vi "MIU_Control_v1.3.vi"() -> ()   [LabVIEW 2010]
uses:
  <vilib>/Utility/error.llb/DialogType.ctl
  <vilib>/Instr/_visa.llb/VISA Configure Serial Port (Instr).vi
  <vilib>/Analysis/NI_AALPro.lvlib
panel:
  in  "Tab Control":T1(tab)=enum."Concentrations"
  in  "Serial Read Port":refnum<visa-resource-name>="COM5"
  in  "data bits":u16=8 min=5 max=8 step=1
  in  "parity":u16(ring) items=["None", "Odd", "Even", "Mark", "Space"]
  in  "stop bits":u16(ring)=10 items=["1.0"=10, "1.5"=15, "2.0"=20]
  in  "flow control":u16(ring) items=["None"=0, "XON/XOFF"=1, "RTS/CTS"=2, "DTR/DSR"=4]
  in  "delay before read (ms)":u32=500
  in  "byte count":u32=500
  out "Incoming Serial String":string="    02/28/13 05:18:49.492,    3.20644e-01,    0.00000e+00,    3.33105e-01,    0.00000e+00,    5.19723e+02,    0.00000e+00,    3.20811e-01,    0.00000e+00,    3.33278e-01,    0.00000e+00,    8.02680e+01,    0.00000e+00,    3.33389e+01,    0.00000e+00,    2.71783e+01,    0.00000e+00,    3.55973e-01,    0.00000e+00,    6.31022e-01,    0.00000e+00,    1.95007e+00,    0.00000e+00,              3\n"
  out "Time":string="05:18:49.492"
  out "Date":string="02/28/13"
  out "return count":u32=394
  in  "Instrument baud rate (9600)":u32=9600
  in  "Control Port":refnum<visa-resource-name>="COM4"
  in  "Control baud rate":u32=9600
  out "N2O is FLAT":bool
  out "Rolling CO Slope Fit":cluster{i32[], "Best Linear Fit":dbl[]}[](graph)=[{[0, 1, 2, 3, 4, 5, 6, 7, 8, 9, 10, 11, 12, 13, 14, 15, 16, 17, 18, 19], "Best Linear Fit"=[0.320611, 0.320505, 0.320476, 0.3208, 0.320926, 0.320701, 0.320587, 0.320889, 0.320914, 0.320439, 0.3209, 0.320794, 0.320847, 0.320592, 0.320735, 0.32085, 0.320821, 0.320729, 0.320589, 0.320309]}, {[0, 1, 2, 3, 4, 5, 6, 7, 8, 9, 10, 11, 12, 13, 14, 15, 16, 17, 18, 19], "Best Linear Fit"=[0.32070674285714285, 0.3207061067669173, 0.3207054706766917, 0.32070483458646615, 0.3207041984962406, 0.32070356240601505, 0.32070292631578945, 0.3207022902255639, 0.32070165413533835, 0.3207010180451128, 0.3207003819548872, 0.32069974586466166, 0.3206991097744361, 0.32069847368421056, 0.32069783759398496, 0.3206972015037594, 0.32069656541353386, 0.32069592932330826, 0.3206952932330827, 0.32069465714285716]}]
  out "CO":dbl(graph)=0.320644
  out "N2O":dbl(graph)=0.333105
  out "H2O":dbl(graph)=519.723
  out "CO PPM":string=" 3.20644e-01"
  out "N2O PPM":string="3.33105e-01"
  out "H2O PPM":string="5.19723e+02"
  in  "Points to Average":i32=30
  out "CO Slope":dbl=-6.360902255623756e-07
  out "Rolling N2O Slope Fit 2":cluster{i32[], "Best Linear Fit":dbl[]}[](graph)=[{[0, 1, 2, 3, 4, 5, 6, 7, 8, 9, 10, 11, 12, 13, 14, 15, 16, 17, 18, 19], "Best Linear Fit"=[0.333232, 0.332975, 0.333256, 0.333094, 0.333062, 0.3332, 0.332763, 0.333281, 0.333155, 0.333115, 0.333375, 0.33321, 0.333348, 0.33294, 0.333468, 0.333464, 0.333003, 0.333373, 0.33336, 0.333239]}, {[0, 1, 2, 3, 4, 5, 6, 7, 8, 9, 10, 11, 12, 13, 14, 15, 16, 17, 18, 19], "Best Linear Fit"=[0.33308077142857145, 0.33309286390977444, 0.3331049563909775, 0.33311704887218047, 0.3331291413533835, 0.3331412338345865, 0.3331533263157895, 0.3331654187969925, 0.3331775112781955, 0.33318960375939854, 0.33320169624060153, 0.3332137887218045, 0.33322588120300756, 0.33323797368421054, 0.3332500661654135, 0.33326215864661657, 0.33327425112781955, 0.3332863436090226, 0.3332984360902256, 0.33331052857142857]}]
  out "N2O Slope":dbl=1.209248120300707e-05
  in  "N2O Low Limit":dbl=-1e-05
  in  "CO High Limit":dbl=1e-05
  out "CO is FLAT":bool
  in  "CO Low Limit":dbl=-1e-05
  in  "N2O High Limit":dbl=1e-05
  out "Switch Valve":bool
  out "Boolean":bool
  in  "Manually Switch Valves":bool=TRUE
  in  "Valve to switch":dbl=1.0 min=0.0 max=16.0 step=1.0
  in  "stop":bool
  in  "switch delay":dbl=15.0
  out "Valve Counter":dbl=1.0
  in  "Num Bottles":dbl=3.0
  out "CELL TEMP":string="3.33389e+01"
  out "CELL TEMPERATURE":dbl(graph)=33.3389
  out "AMBIENT TEMPERATURE":dbl(graph)=27.1783
  out "AMBIENT TEMP":string="2.71783e+01"
  out "AIN5":dbl(graph)=0.631022
  out "SUPERCOOL TEMP":string="6.31022e-01"
  out "LINE LOCK":dbl(graph)=0.355973
  out "LINELOCK - LASER CONTROL VOLTAGE":string="3.55973e-01"
  out "PRESSURE":dbl(graph)=80.268
  out "PRESSURE 2":string="8.02680e+01"
  out "CO DRY 2":dbl(graph)=0.320811
  out "N2O DRY":dbl(graph)=0.333278
  out "CO DRY":string="3.20811e-01"
  out "N2O DRY 2":string="3.33278e-01"
  # "Automatic Linearization"
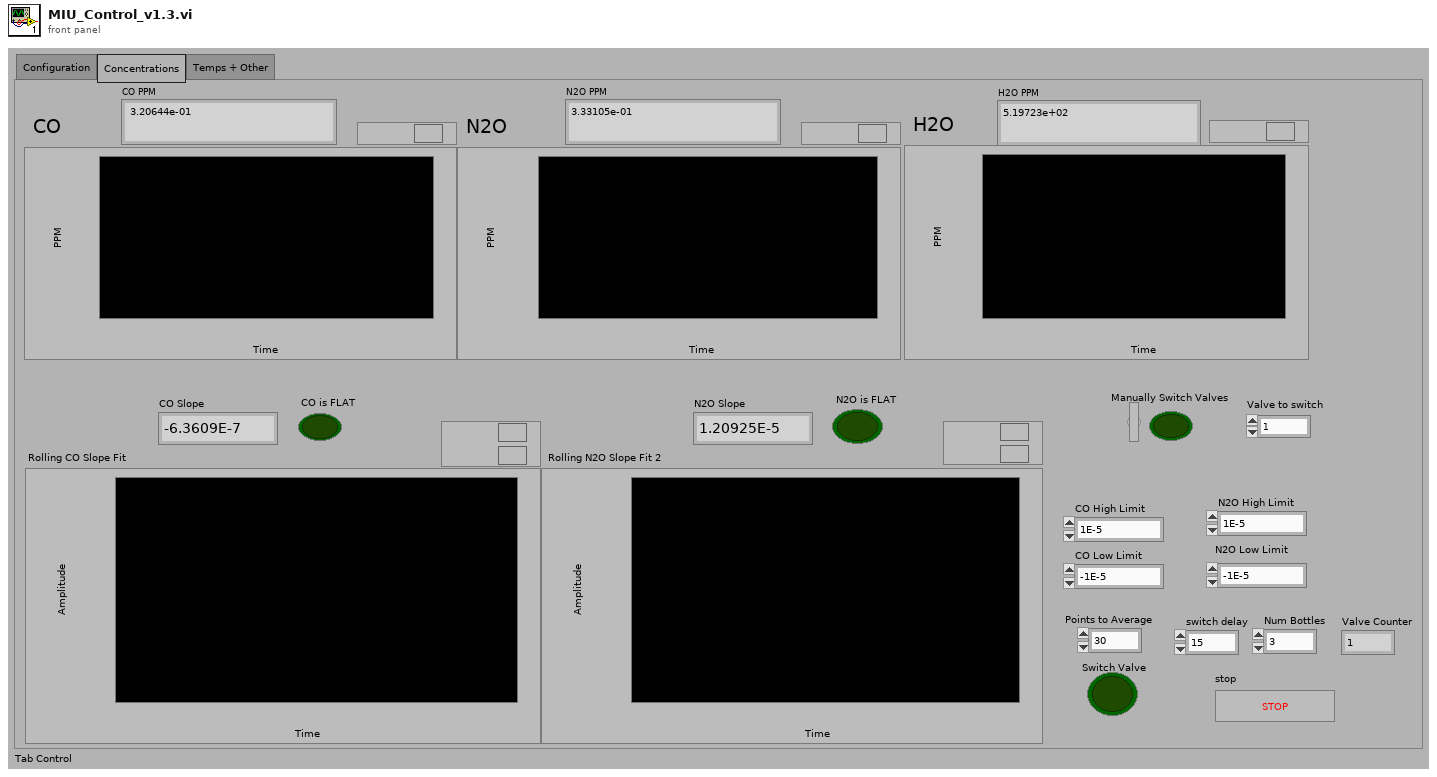
[diagram p1: front panel]
types:
  T1 = enum32{"Configuration", "Concentrations", "Temps + Other"}
  T2 = typedef "DialogType.ctl" = u16
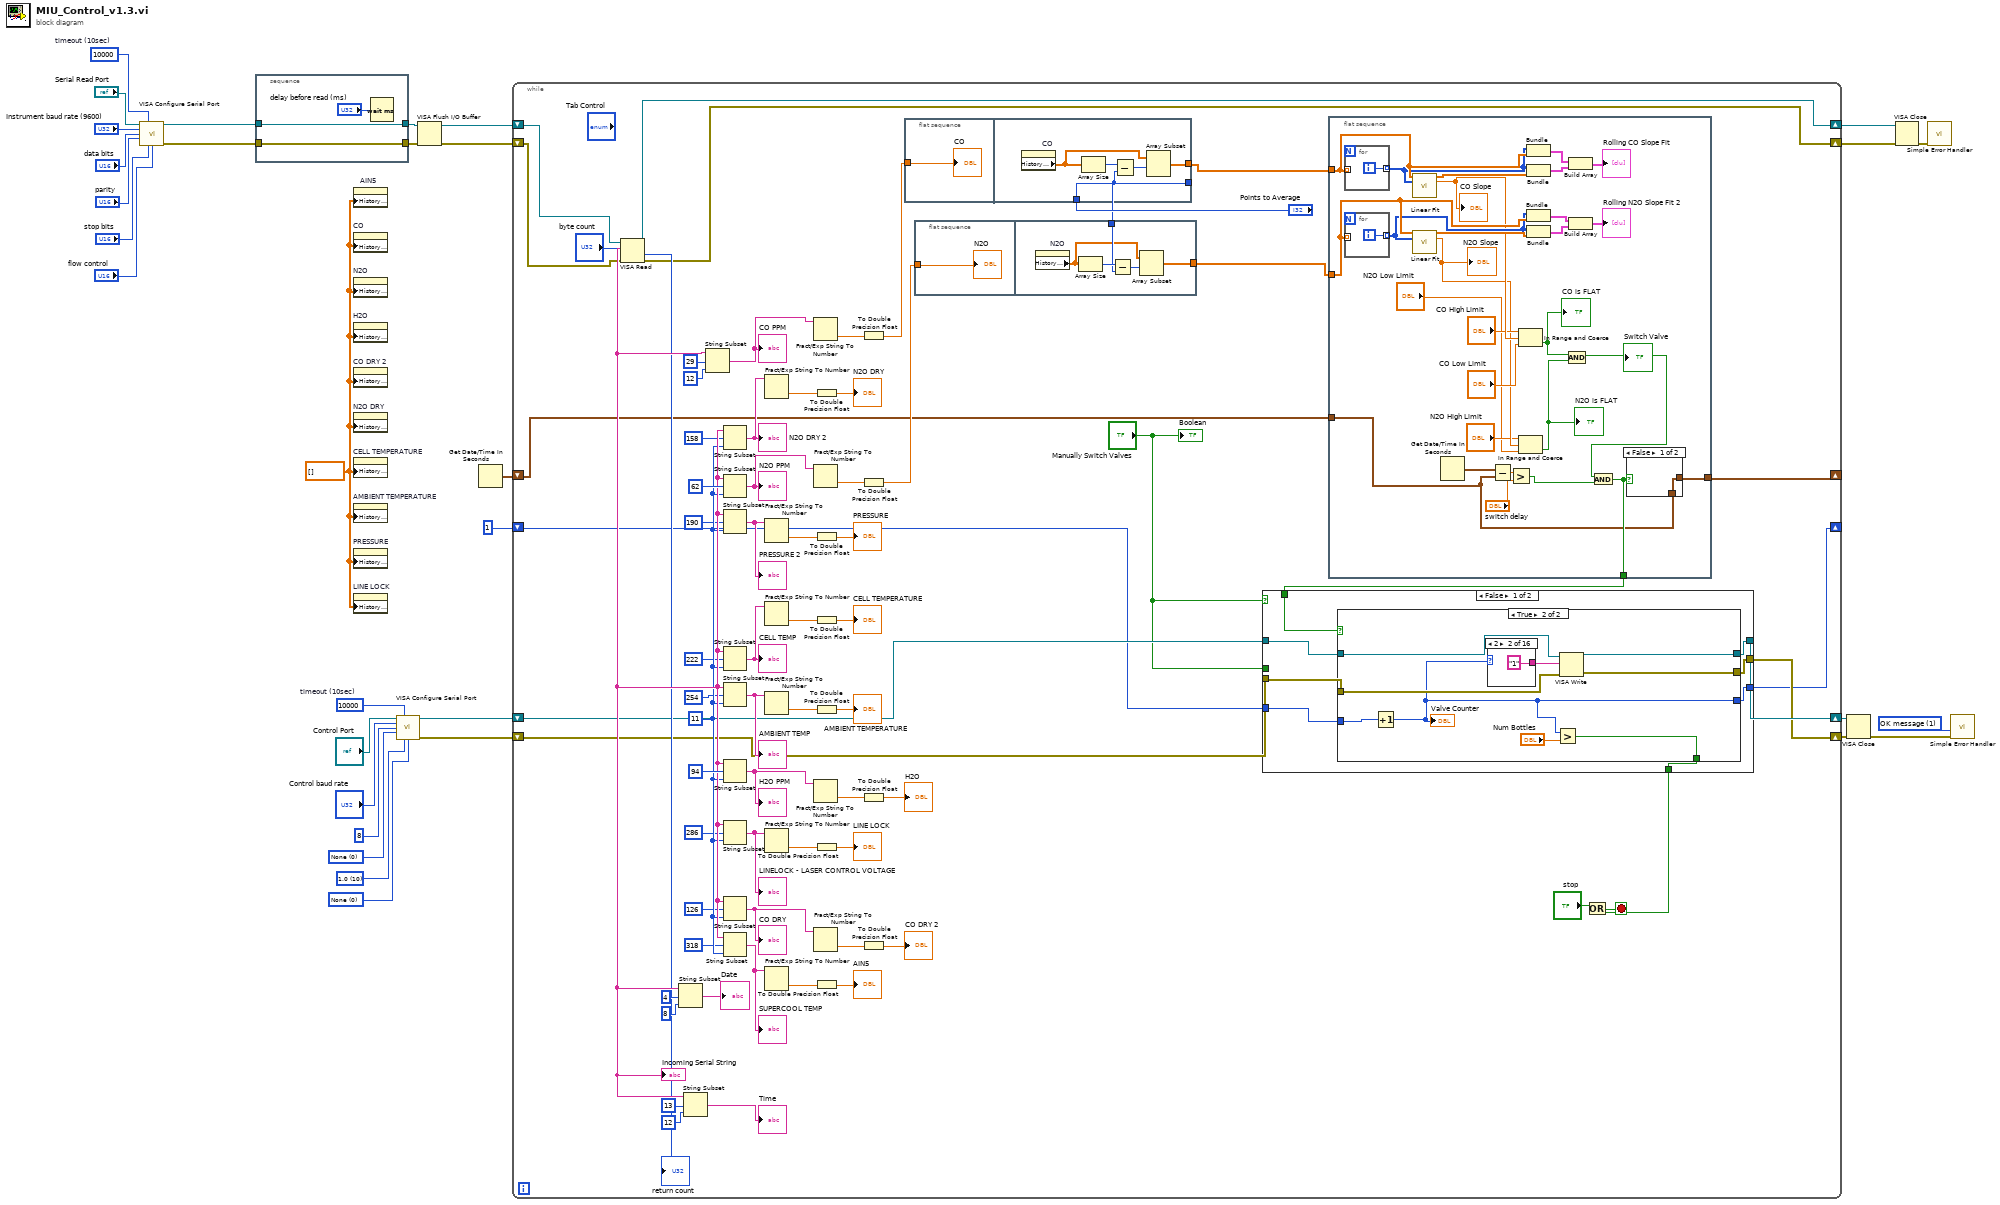
[diagram p0: block diagram]
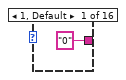
[diagram p3: hidden frame]
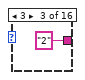
[diagram p4: hidden frame]
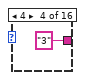
[diagram p5: hidden frame]
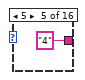
[diagram p6: hidden frame]
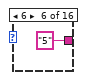
[diagram p7: hidden frame]
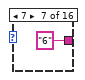
[diagram p8: hidden frame]
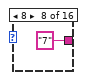
[diagram p9: hidden frame]
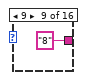
[diagram p10: hidden frame]
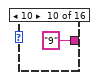
[diagram p11: hidden frame]
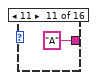
[diagram p12: hidden frame]
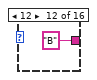
[diagram p13: hidden frame]
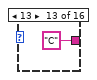
[diagram p14: hidden frame]
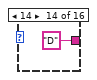
[diagram p15: hidden frame]
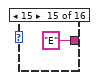
[diagram p16: hidden frame]
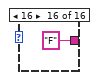
[diagram p17: hidden frame]
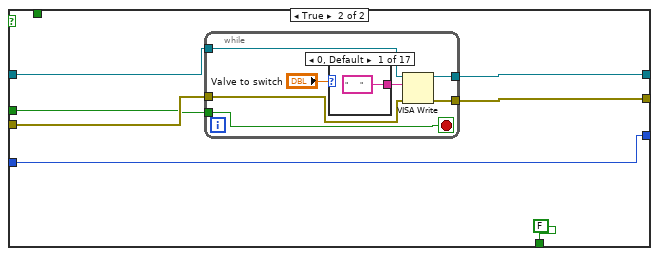
[diagram p18: hidden frame]
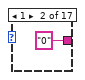
[diagram p19: hidden frame]
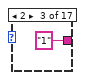
[diagram p20: hidden frame]
diagram:
  w7 = T2 1 items=["no dialog", "OK message", "continue or stop message", "OK message + warnings", "continue/stop + warnings"] ("type of dialog (OK msg:1)")
  w11 = u16 0 items=["None"=0, "XON/XOFF"=1, "RTS/CTS"=2, "DTR/DSR"=4] ("flow control")
  w12 = u16 10 items=["1.0"=10, "1.5"=15, "2.0"=20] ("stop bits")
  w14 = u16 0 items=["None", "Odd", "Even", "Mark", "Space"] ("parity")
  w13 = u32 10000  # timeout (10sec)
  w17 = dbl[] [] ("History Data")
  w29 = u32 10000  # timeout (10sec)
  n1 = call-poly "VISA Configure Serial Port"("VISA resource name"="Serial Read Port", "timeout (10sec)"=w29, "baud rate (9600)"="Instrument baud rate (9600)", "data bits (8)"="data bits", "parity (0:none)"="parity", "stop bits (10: 1 bit)"="stop bits", "flow control (0:none)"="flow control") -> ("VISA resource name out"=w24:refnum<visa-resource-name>, "error out"=w25:errorcluster)  [unwired: 2 in, 5 out]
  n2 = stacked-sequence {
    tunnel: w25 -> [w35]
    tunnel: [w35] -> w18
    tunnel: w24 -> [w34]
    tunnel: [w34] -> w19
    frame #0 {
      n3 = Wait (ms)(milliseconds to wait="delay before read (ms)") -> ()  [unwired: 1 out]
    }
  }
  n4 = property on="AIN5" class="WFChart (strict)"("History Data"=w17) -> ()  [unwired: 2 in, 2 out]
  n5 = property on="CO" class="WFChart (strict)"("History Data"=w17) -> ()  [unwired: 2 in, 2 out]
  n6 = property on="N2O" class="WFChart (strict)"("History Data"=w17) -> ()  [unwired: 2 in, 2 out]
  n7 = property on="H2O" class="WFChart (strict)"("History Data"=w17) -> ()  [unwired: 2 in, 2 out]
  n8 = property on="CO DRY 2" class="WFChart (strict)"("History Data"=w17) -> ()  [unwired: 2 in, 2 out]
  n9 = property on="N2O DRY" class="WFChart (strict)"("History Data"=w17) -> ()  [unwired: 2 in, 2 out]
  n10 = property on="CELL TEMPERATURE" class="WFChart (strict)"("History Data"=w17) -> ()  [unwired: 2 in, 2 out]
  n11 = property on="AMBIENT TEMPERATURE" class="WFChart (strict)"("History Data"=w17) -> ()  [unwired: 2 in, 2 out]
  n12 = property on="PRESSURE" class="WFChart (strict)"("History Data"=w17) -> ()  [unwired: 2 in, 2 out]
  n13 = property on="LINE LOCK" class="WFChart (strict)"("History Data"=w17) -> ()  [unwired: 2 in, 2 out]
  n14 = call-poly "VISA Configure Serial Port"("VISA resource name"="Control Port", "timeout (10sec)"=w13, "baud rate (9600)"="Control baud rate", "data bits (8)"=u16 8 ("data bits"), "parity (0:none)"=w14, "stop bits (10: 1 bit)"=w12, "flow control (0:none)"=w11) -> ("VISA resource name out"=w6:refnum<visa-resource-name>, "error out"=w5:errorcluster)  [unwired: 2 in, 5 out]
  n15 = VISA Flush I/O Buffer(VISA resource name=w19, error in (no error)=w18) -> (VISA resource name out=w21:refnum<visa-resource-name>, error out=w20:errorcluster)  [unwired: 1 in]
  n16 = Get Date/Time In Seconds() -> (seconds since 1Jan1904=w1:timestamp)
  n17 = while {
    shift-right: [w51] -> w4
    shift-left: w6 -> [w49]
    shift-right: [w50] -> w3
    shift-left: w5 -> [w48]
    shift-right: [w101] -> w23
    shift-left: w21 -> [w42]
    shift-right: [w60] -> w22
    shift-left: w20 -> [w43]
    shift-right: [w39] -> _
    shift-left: 1 -> [w40]
    shift-right: [w36] -> _
    shift-left: w1 -> [w38]
    stop <- w54 stop-if-true
    w70 = 11 ("offset (0)")
    n18 = VISA Read(VISA resource name=w42, byte count="byte count", error in (no error)=w43) -> (VISA resource name out=w101:refnum<visa-resource-name>, read buffer=w71:string, return count=→"return count":u32, error out=w60:errorcluster)
    "Incoming Serial String" <- w71
    n19 = String Subset(string=w71, offset (0)=4, length (rest)=8 ("length (rest)")) -> (substring=→"Date":string)
    n20 = String Subset(string=w71, offset (0)=13, length (rest)=12 ("length (rest)")) -> (substring=→"Time":string)
    n21 = String Subset(string=w71, offset (0)=29, length (rest)=12 ("length (rest)")) -> (substring=w96:string)
    "CO PPM" <- w96
    n22 = String Subset(string=w71, offset (0)=158, length (rest)=w70) -> (substring=w82:string)
    "N2O DRY 2" <- w82
    n23 = String Subset(string=w71, offset (0)=62, length (rest)=w70) -> (substring=w95:string)
    "N2O PPM" <- w95
    n24 = String Subset(string=w71, offset (0)=190, length (rest)=w70) -> (substring=w81:string)
    "PRESSURE 2" <- w81
    n25 = String Subset(string=w71, offset (0)=222, length (rest)=w70) -> (substring=w80:string)
    "CELL TEMP" <- w80
    n26 = String Subset(string=w71, offset (0)=254, length (rest)=w70) -> (substring=w74:string)
    "AMBIENT TEMP" <- w74
    n27 = String Subset(string=w71, offset (0)=94, length (rest)=w70) -> (substring=w94:string)
    "H2O PPM" <- w94
    n28 = String Subset(string=w71, offset (0)=286, length (rest)=w70) -> (substring=w73:string)
    "LINELOCK - LASER CONTROL VOLTAGE" <- w73
    n29 = String Subset(string=w71, offset (0)=126, length (rest)=w70) -> (substring=w83:string)
    "CO DRY" <- w83
    n30 = String Subset(string=w71, offset (0)=318, length (rest)=w70) -> (substring=w72:string)
    "SUPERCOOL TEMP" <- w72
    n31 = Fract/Exp String To Number(string=w82) -> (number=w88:dbl)  [unwired: 3 in, 1 out]
    n32 = Fract/Exp String To Number(string=w81) -> (number=w86:dbl)  [unwired: 3 in, 1 out]
    n33 = Fract/Exp String To Number(string=w80) -> (number=w84:dbl)  [unwired: 3 in, 1 out]
    n34 = Fract/Exp String To Number(string=w74) -> (number=w78:dbl)  [unwired: 3 in, 1 out]
    n35 = Fract/Exp String To Number(string=w73) -> (number=w76:dbl)  [unwired: 3 in, 1 out]
    n36 = Fract/Exp String To Number(string=w72) -> (number=w75:dbl)  [unwired: 3 in, 1 out]
    n37 = Fract/Exp String To Number(string=w96) -> (number=w93:dbl)  [unwired: 3 in, 1 out]
    n38 = Fract/Exp String To Number(string=w95) -> (number=w59:dbl)  [unwired: 3 in, 1 out]
    n39 = Fract/Exp String To Number(string=w94) -> (number=w92:dbl)  [unwired: 3 in, 1 out]
    n40 = Fract/Exp String To Number(string=w83) -> (number=w90:dbl)  [unwired: 3 in, 1 out]
    n41 = To Double Precision Float(number=w88) -> (double precision float=→"N2O DRY":dbl)
    n42 = To Double Precision Float(number=w86) -> (double precision float=→"PRESSURE":dbl)
    n43 = To Double Precision Float(number=w84) -> (double precision float=→"CELL TEMPERATURE":dbl)
    n44 = To Double Precision Float(number=w78) -> (double precision float=→"AMBIENT TEMPERATURE":dbl)
    n45 = To Double Precision Float(number=w76) -> (double precision float=→"LINE LOCK":dbl)
    n46 = To Double Precision Float(number=w75) -> (double precision float=→"AIN5":dbl)
    n47 = To Double Precision Float(number=w93) -> (double precision float=w53:dbl)
    n48 = To Double Precision Float(number=w59) -> (double precision float=w52:dbl)
    n49 = To Double Precision Float(number=w92) -> (double precision float=→"H2O":dbl)
    n50 = To Double Precision Float(number=w90) -> (double precision float=→"CO DRY 2":dbl)
    n51 = flat-sequence {
      tunnel: w53 -> [w214]
      tunnel: [w216] -> w45
      tunnel: "Points to Average" -> [w215]
      tunnel: [w215] -> w57
      frame #0 {
        "CO" <- w214
      }
      frame #1 {
        n52 = property on="CO" class="WFChart (strict)"() -> ("History Data"=w217:dbl[])  [unwired: 2 in, 2 out]
        n53 = Array Size(array=w217) -> (size(s)=w218:i32)
        n54 = Subtract(x=w218, y=w215) -> (x-y=w219:i32)
        n55 = Array Subset(array=w217, index=w219) -> (w216:dbl[])  [unwired: 1 in]
      }
    }
    n56 = flat-sequence {
      tunnel: w52 -> [w208]
      tunnel: w57 -> [w211]
      tunnel: [w209] -> w46
      frame #0 {
        "N2O" <- w208
      }
      frame #1 {
        n57 = property on="N2O" class="WFChart (strict)"() -> ("History Data"=w210:dbl[])  [unwired: 2 in, 2 out]
        n58 = Array Size(array=w210) -> (size(s)=w212:i32)
        n59 = Subtract(x=w212, y=w211) -> (x-y=w213:i32)
        n60 = Array Subset "Array Subset"(array=w210, index=w213) -> (w209:dbl[])  [unwired: 1 in]
      }
    }
    n61 = case shown="False" "Manually Switch Valves" {
      tunnel: [w115 w151] -> w51
      tunnel: [w114 w150] -> w50
      tunnel: w49 -> [w113 w149]
      tunnel: w48 -> [w112 w148]
      tunnel: "Manually Switch Valves" -> [_ w147]
      tunnel: [w111 FALSE] -> w41
      tunnel: w40 -> [w110 w145]
      tunnel: w37 -> [w109 _]
      tunnel: [w108 w145] -> w39
      frame False {
        n62 = case shown="True" w109 {
          selector: w109 -> [w117 _]
          tunnel: [w119 w126] -> w115
          tunnel: [w118 w127] -> w114
          tunnel: w113 -> [w119 w125]
          tunnel: w112 -> [w118 w124]
          tunnel: [w117 w122] -> w111
          tunnel: w110 -> [w116 w121]
          tunnel: [w116 w120] -> w108
          frame False {
          }
          frame True {
            n63 = Increment(x=w121) -> (x+1=w120:i32)
            "Valve Counter" <- w120
            n64 = case shown="2" w120 {
              tunnel: ["0" "1" "2" "3" "4" "5" "6" "7" "8" "9" "A" "B" "C" "D" "E" "F"] -> w128
              frame 1, Default {
              }
              frame 2 {
              }
              frame 3 {
              }
              frame 4 {
              }
              frame 5 {
              }
              frame 6 {
              }
              frame 7 {
              }
              frame 8 {
              }
              frame 9 {
              }
              frame 10 {
              }
              frame 11 {
              }
              frame 12 {
              }
              frame 13 {
              }
              frame 14 {
              }
              frame 15 {
              }
              frame 16 {
              }
            }
            n65 = Greater?(x=w120, y="Num Bottles") -> (0:w122:bool)
            n66 = VISA Write(VISA resource name=w125, write buffer=w128, error in (no error)=w124) -> (VISA resource name out=w126:refnum<visa-resource-name>, error out=w127:errorcluster)  [unwired: 1 out]
          }
        }
      }
      frame True {
        n67 = while {
          tunnel: [w156] -> w151
          tunnel: [w155] -> w150
          tunnel: w149 -> [w154]
          tunnel: w148 -> [w153]
          tunnel: w147 -> [w152]
          stop <- w152 stop-if-true
          n68 = case shown="0, Default" "Valve to switch" {
            tunnel: ["      " "0" "1" "2" "3" "4" "5" "6" "7" "8" "9" "A" "B" "C" "D" "E" "F"] -> w158
            frame 0, Default {
            }
            frame 1 {
            }
            frame 2 {
            }
            frame 3 {
            }
            frame 4 {
            }
            frame 5 {
            }
            frame 6 {
            }
            frame 7 {
            }
            frame 8 {
            }
            frame 9 {
            }
            frame 10 {
            }
            frame 11 {
            }
            frame 12 {
            }
            frame 13 {
            }
            frame 14 {
            }
            frame 15 {
            }
            frame 16 {
            }
          }
          n69 = VISA Write(VISA resource name=w154, write buffer=w158, error in (no error)=w153) -> (VISA resource name out=w156:refnum<visa-resource-name>, error out=w155:errorcluster)  [unwired: 1 out]
        }
      }
    }
    n70 = flat-sequence {
      tunnel: w45 -> [w203]
      tunnel: w46 -> [w202]
      tunnel: w38 -> [w176]
      tunnel: [w178] -> w37
      tunnel: [w177] -> w36
      frame #0 {
        n71 = for {
          tunnel: [w207] -> w201 mode=indexing
          tunnel: w203 -> [_] mode=indexing
          i -> [w207]
        }
        n72 = for {
          tunnel: [w206] -> w196 mode=indexing
          tunnel: w202 -> [_] mode=indexing
          i -> [w206]
        }
        n73 = call <vilib>:"Linear Fit.vi"("Y"=w203, "X"=w201) -> ("Best Linear Fit"=w200:dbl[], "slope"=w191:dbl)  [unwired: 9 in, 3 out]
        "CO Slope" <- w191
        n74 = call <vilib>:"Linear Fit.vi"("Y"=w202, "X"=w196) -> ("Best Linear Fit"=w195:dbl[], "slope"=w188:dbl)  [unwired: 9 in, 3 out]
        "N2O Slope" <- w188
        n75 = Get Date/Time In Seconds() -> (seconds since 1Jan1904=w183:timestamp)
        n76 = Subtract(x=w183, y=w176) -> (x-y=w182:dbl)
        n77 = Greater?(x=w182, y="switch delay") -> (0:w180:bool)
        n78 = In Range and Coerce(upper limit="CO High Limit", x=w191, lower limit="CO Low Limit") -> (In Range?=w185:bool)  [unwired: 1 out]
        "CO is FLAT" <- w185
        n79 = In Range and Coerce(upper limit="N2O High Limit", x=w188, lower limit="N2O Low Limit") -> (In Range?=w184:bool)  [unwired: 1 out]
        "N2O is FLAT" <- w184
        n80 = Bundle(w201, w203) -> (w199:cluster{i32[], dbl[]})  [unwired: 1 in]
        n81 = Bundle(w201, "Best Linear Fit"=w200) -> (w198:cluster{i32[], "Best Linear Fit":dbl[]})  [unwired: 1 in]
        n82 = Bundle(w196, w202) -> (w194:cluster{i32[], dbl[]})  [unwired: 1 in]
        n83 = Bundle(w196, "Best Linear Fit"=w195) -> (w193:cluster{i32[], "Best Linear Fit":dbl[]})  [unwired: 1 in]
        n84 = And(x=w185, y=w184) -> (x .and. y?=w179:bool)
        "Switch Valve" <- w179
        n85 = Build Array(w199, w198) -> (→"Rolling CO Slope Fit":cluster{i32[], "Best Linear Fit":dbl[]}[])
        n86 = Build Array(w194, w193) -> (→"Rolling N2O Slope Fit 2":cluster{i32[], "Best Linear Fit":dbl[]}[])
        n87 = And(x=w179, y=w180) -> (x .and. y?=w178:bool)
        n88 = case shown="False" w178 {
          tunnel: [w204 w205] -> w177
          tunnel: w176 -> [w204 _]
          frame False {
          }
          frame True {
            n89 = Get Date/Time In Seconds() -> (seconds since 1Jan1904=w205:timestamp)
          }
        }
      }
    }
    n90 = Or(x="stop", y=w41) -> (x .or. y?=w54:bool)
    "Boolean" <- "Manually Switch Valves"
  }
  n91 = VISA Close(VISA resource name=w4, error in (no error)=w3) -> (error out=w9:errorcluster)
  n92 = VISA Close(VISA resource name=w23, error in (no error)=w22) -> (error out=w31:errorcluster)
  n93 = call <vilib>:"Simple Error Handler.vi"("error in (no error)"=w31) -> ()  [unwired: 1 in, 8 out]
  n94 = call <vilib>:"Simple Error Handler.vi"("type of dialog (OK msg:1)"=w7, "error in (no error)"=w9) -> ()  [unwired: 8 out]
